vi "Write LSEOutput.vi"(8 "error in (no error)":errorcluster, 10 "LSEOutput":T1={"SystemVoltagesRef"=[], "Vestimate"=[], "LSEConfig"={"NoiseVariance"=0.001, "IEEESystem"=5, "PMULocations"=[1], "Vindex"=0, "Iindex"=3, "DynamicRef"=""}, "Bus"=[]}, 11 "VisualizeAppLSE in":refnum<class "VisualizeAppLSE.lvclass">) -> (0 "error out":errorcluster, 3 "VisualizeAppLSE out":refnum<class "VisualizeAppLSE.lvclass">)   [LabVIEW 2014, in "Visualization.lvlib" / "VisualizeAppLSE.lvclass"]
uses:
  VisualizeAppLSE.lvclass
  Modules/AppPlugins/LSEPlugin/PublicAPI/Typedefs/LSEOutput.ctl
  Modules/AppPlugins/LSEPlugin/PublicAPI/Typedefs/LSEConfig.ctl
  VisualizeAppLSE.lvclass/VisualizeAppLSE.ctl
  Modules/AppPlugins/LSEPlugin/LSEPlugin.lvclass
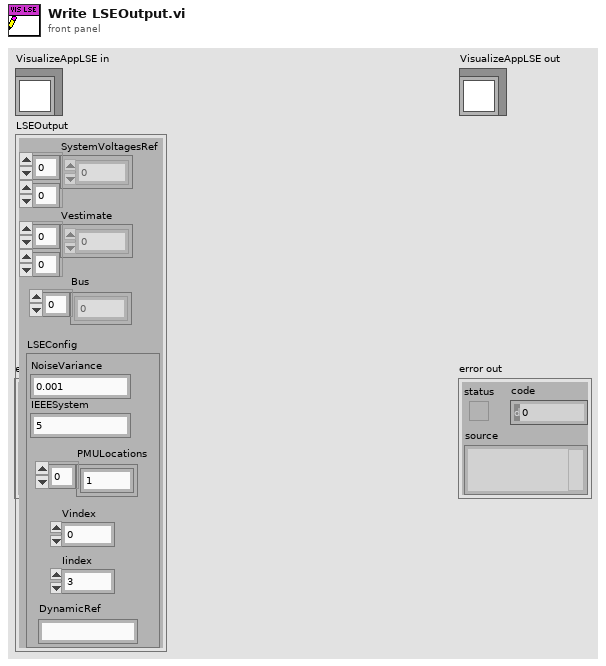
[diagram p1: front panel]
types:
  T1 = typedef "AppPlugins.lvlib/LSEPlugin.lvclass/LSEOutput.ctl" = cluster{"SystemVoltagesRef":cdb[][], "Vestimate":cdb[][], "LSEConfig":T2, "Bus":dbl[]}
  T2 = typedef "AppPlugins.lvlib/LSEPlugin.lvclass/LSEConfig.ctl" = cluster{"NoiseVariance":dbl, "IEEESystem":u32, "PMULocations":u32[], "Vindex":i32, "Iindex":i32, "DynamicRef":string}
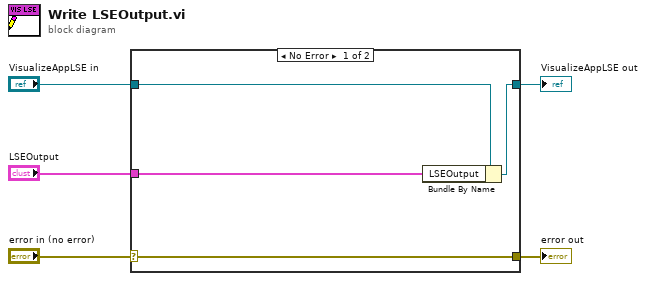
[diagram p0: block diagram]
diagram:
  n1 = case shown="No Error" "error in (no error)" {
    selector: "error in (no error)" -> [w9 w10]
    tunnel: [w9 w10] -> w4
    tunnel: [w7 w11] -> w2
    tunnel: "VisualizeAppLSE in" -> [w8 w11]
    tunnel: "LSEOutput" -> [w6 _]
    frame No Error {
      n2 = Bundle By Name(cluster=w8, "LSEOutput"=w6) -> (w7:refnum<class "VisualizeAppLSE.lvclass">)
    }
    frame Error {
    }
  }
  "error out" <- w4
  "VisualizeAppLSE out" <- w2
